vi "Limit Row Count in Table.vi"(9 "Insert":string[](array[string]), 10 "Data_In":string[][](array[string]), 11 "MaxDataQueue":u16=5) -> (2 "Data_out":string[][](array[string]))   [LabVIEW 2019]
uses:
  <userlib>/_OpenG.lib/array/array.llb/Reverse 2D Array (String)__ogtk.vi
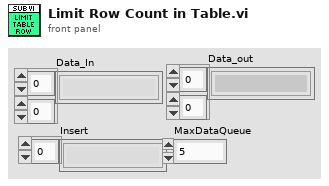
[diagram p1: front panel]
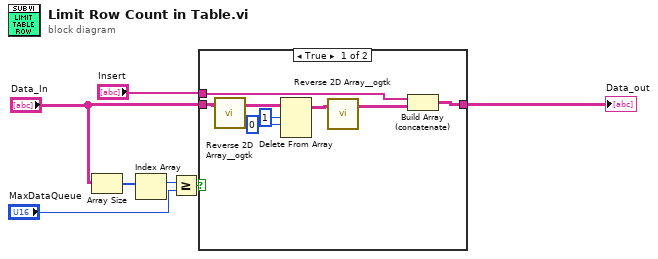
[diagram p0: block diagram]
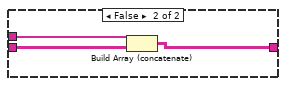
[diagram p2: hidden frame]
diagram:
  n1 = Array Size(array="Data_In") -> (size(s)=w5:i32[])
  n2 = Index Array(array=w5) -> (element=w2:i32)  [unwired: 1 in]
  n3 = Greater Or Equal?(x=w2, y="MaxDataQueue") -> (x >= y?=w3:bool)
  n4 = case shown="True" w3 {
    tunnel: [w15 w18] -> w6
    tunnel: "Data_In" -> [w12 w17]
    tunnel: "Insert" -> [w8 w16]
    frame True {
      n5 = call-poly <userlib>:"Reverse 2D Array__ogtk.vi"("Array"=w12) -> ("Reversed Array"=w11:string[][])  [unwired: 2 in]
      n6 = Delete From Array(array=w11, length=1, index (row)=0 ("index")) -> (array with subset deleted=w10:string[][])  [unwired: 1 in, 1 out]
      n7 = call-poly <userlib>:"Reverse 2D Array__ogtk.vi"("Array"=w10) -> ("Reversed Array"=w9:string[][])  [unwired: 2 in]
      n8 = Build Array (concatenate)(w8, w9) -> (w15:string[][])
    }
    frame False {
      n9 = Build Array (concatenate)(w16, w17) -> (w18:string[][])
    }
  }
  "Data_out" <- w6
